vi "Configure Instrument.vi"(6 "Common Mode Reduction (T: On)":bool=TRUE, 7 "Monitor Output (7: VAD Control)":u16(ring)=7 items=["Off", "CS NEG", "CS POS", "VCM NEG", "VCM POS", "VDIF", "VAD-Measurement", "VAD - Control"], 8 "error in (no error)":errorcluster, 9 "Excitation Frequency (2: 13.7 Hz)":u16(ring)=2 items=["9.8 Hz"=1, "13.7 Hz"=2, "16.2 Hz"=3], 10 "Channel (0: Measurement Input)":u16(ring) items=["Measurement Input", "Control Input (A)"], 11 "VISA resource name":refnum<visa-resource-name>) -> (0 "error out":errorcluster, 3 "VISA resource name out":refnum<visa-resource-name>)   [LabVIEW 2018, in "Lake Shore 372.lvlib"]
doc: "Configures the instrument set up. Parameters configured are;\nExcitation Frequency, Common Mode Reduction, and Monitor Output.\nThe commands used are <B>FREQ</B>, <B>CMR</B>, and <B>MONITOR</B>.\n\nNote:\nFrequency takes several seconds to complete."
uses:
  Lake Shore 372.lvlib
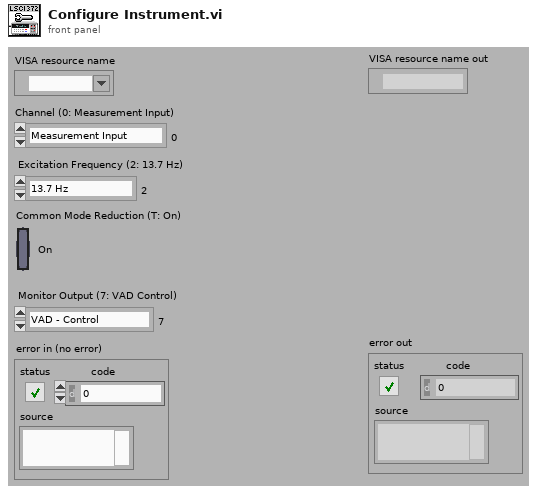
[diagram p1: front panel]
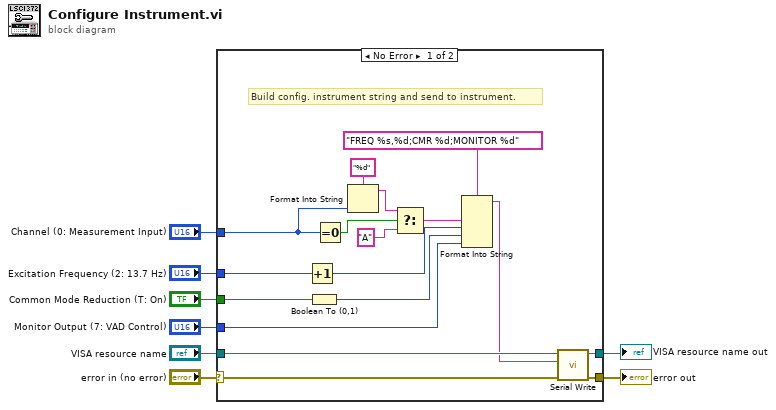
[diagram p0: block diagram]
diagram:
  n1 = case shown="No Error" "error in (no error)" {
    selector: "error in (no error)" -> [w9 w26]
    tunnel: "VISA resource name" -> [w25 w27]
    tunnel: [w24 w26] -> w7
    tunnel: [w23 w27] -> w6
    tunnel: "Excitation Frequency (2: 13.7 Hz)" -> [w22 _]
    tunnel: "Common Mode Reduction (T: On)" -> [w21 _]
    tunnel: "Monitor Output (7: VAD Control)" -> [w17 _]
    tunnel: "Channel (0: Measurement Input)" -> [w11 _]
    frame No Error {
      # "Build config. instrument string and send to instrument."
      n2 = Increment(x=w22) -> (x+1=w19:u16)
      n3 = Boolean To (0,1)(Boolean=w21) -> (0, 1=w18:i16)
      n4 = Equal To 0?(x=w11) -> (x = 0?=w14:bool)
      n5 = Format Into String(format string="%d", w11) -> (resulting string=w12:string)  [unwired: 2 in, 1 out]
      n6 = Select(t=w12, s=w14, f="A" ("format string")) -> (s? t:f=w10:string)
      n7 = Format Into String(format string="FREQ %s,%d;CMR %d;MONITOR %d", w10, w19, w18, w17) -> (resulting string=w16:string)  [unwired: 2 in, 1 out]
      n8 = call "Serial Write.vi"("error in (no error)"=w9, "Write Buffer (\"\")"=w16, "VISA resource name"=w25) -> ("error out"=w24:errorcluster, "VISA resource name out"=w23:refnum<visa-resource-name>)  [unwired: 6 in, 1 out]
    }
    frame Error {
    }
  }
  "error out" <- w7
  "VISA resource name out" <- w6
